vi "Create Name Msg Input.vi"(6 "Name Msg":string, 8 "error in":errorcluster, 9 "Name Library File Path":path, 10 "Active Project":refnum<vi>) -> (0 "error out":errorcluster, 2 "Name Msg IO (Input)":T1)   [LabVIEW 2025, in "_Rescript.lvlib" / "Msg.lvlib" / "Msg.lvclass"]
uses:
  Msg.lvclass
  Name Msg IO.ctl
  Terminal Attributes.ctl
  Attributes.ctl
  IO.ctl
  _Rescript.lvlib
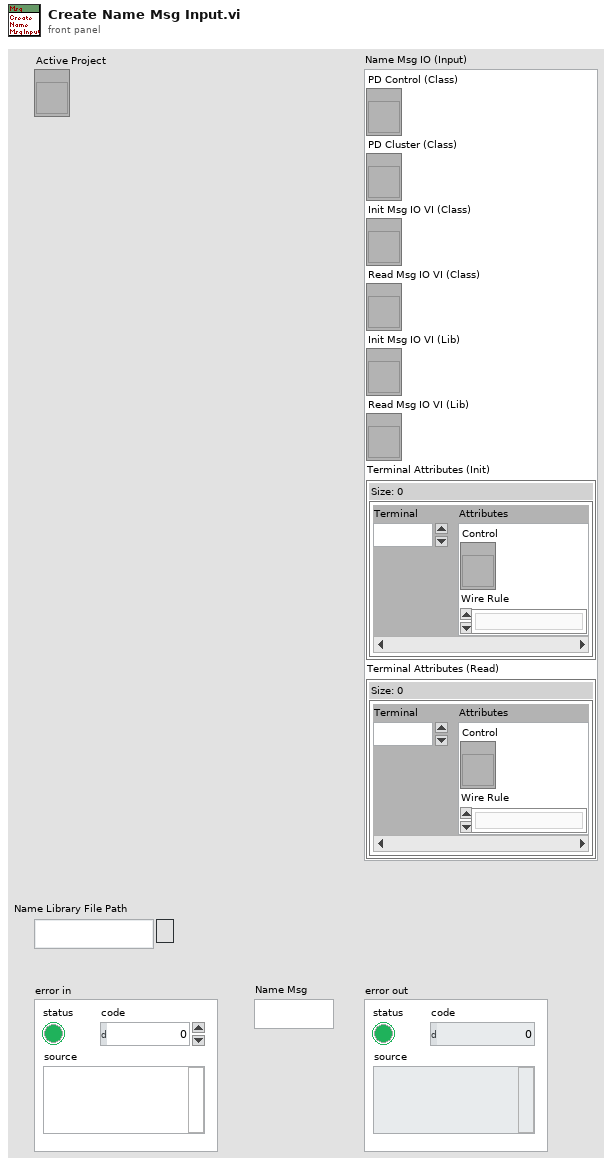
[diagram p1: front panel]
types:
  T1 = typedef "_Rescript.lvlib/Msg.lvlib/Msg.lvclass/Name Msg IO.ctl" = cluster{"PD Control (Class)":refnum<vi>, "PD Cluster (Class)":refnum<vi>, "Init Msg IO VI (Class)":refnum<vi>, "Read Msg IO VI (Class)":refnum<vi>, "Init Msg IO VI (Lib)":refnum<vi>, "Read Msg IO VI (Lib)":refnum<vi>, "Terminal Attributes (Init)":T2, "Terminal Attributes (Read)":T2}
  T2 = typedef "_Rescript.lvlib/Terminal Attributes.ctl" = map{i32, T3}
  T3 = typedef "_Rescript.lvlib/Attributes.ctl" = cluster{"Control":refnum<vi>, "Wire Rule":enum16{"Invalid Wire Rule", "Required", "Recommended", "Optional", "Dynamic Dispatch"}}
  T4 = typedef "_Rescript.lvlib/Msg.lvlib/Msg.lvclass/IO.ctl" = enum16{"Input", "Output"}
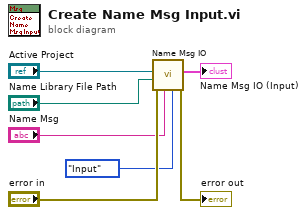
[diagram p0: block diagram]
diagram:
  n1 = call "Name Msg IO.vi"("IO"=IO."Input", "Name Msg"="Name Msg", "error in"="error in", "Name Library File Path"="Name Library File Path", "Active Project"="Active Project") -> ("error out"=→"error out":errorcluster, "Name Msg IO"=→"Name Msg IO (Input)":T1)  [unwired: 5 in]
